vi "Path Keeper_User Find and Write.vi"(7 "Previous location":path, 8 "Error In":errorcluster, 9 "File(f)\nDirectory(t) In":bool, 10 "File / Directory Name In":string, 11 "Refnum In":T1) -> (0 "Error Out":errorcluster, 1 "Valid Path Out":bool, 2 "Path Out":path, 3 "Config Data Out":T1)   [LabVIEW 2015]
uses:
  <vilib>/Utility/config.llb/Config Data RefNum.ctl
  <vilib>/Utility/config.llb/NI_LVConfig.lvlib
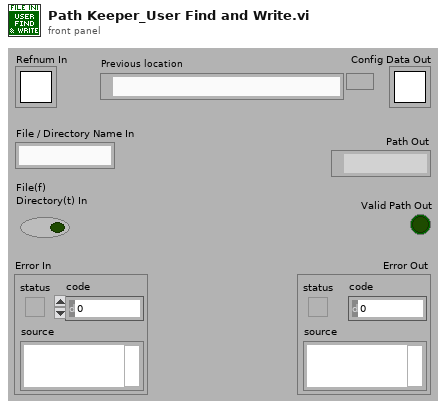
[diagram p1: front panel]
types:
  T1 = typedef "NI_LVConfig.lvlib/Config Data RefNum.ctl" = refnum<k1>
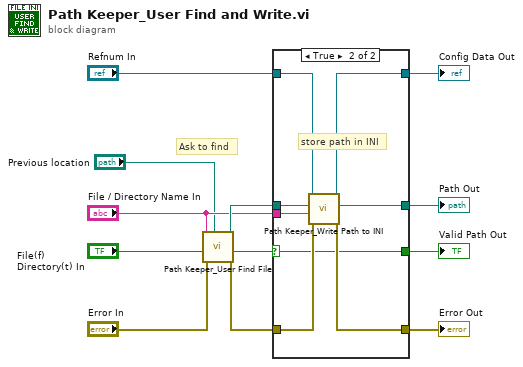
[diagram p0: block diagram]
diagram:
  # "Ask to find"
  n1 = call "Path Keeper_User Find File.vi"("Previous Path"="Previous location", "error In"="Error In", "File(f)\nDirectory(t) In"="File(f)\nDirectory(t) In", "File / Directory Name In"="File / Directory Name In") -> ("error Out"=w8:errorcluster, "Valid Item Out"=w10:bool, "path Out"=w4:path)  [unwired: 5 in]
  n2 = case shown="True" w10 {
    selector: w10 -> [w14 w16]
    tunnel: "File / Directory Name In" -> [_ w23]
    tunnel: w4 -> [_ w22]
    tunnel: "Refnum In" -> [w15 w21]
    tunnel: [w15 w20] -> w6
    tunnel: w8 -> [w13 w19]
    tunnel: [w13 w18] -> w9
    tunnel: [_ w17] -> w11
    tunnel: [w14 w16] -> w12
    frame False {
      # "No Path Found"
    }
    frame True {
      # "store path in INI"
      n3 = call "Path Keeper_Write Path to INI.vi"("Error In"=w19, "File / Directory Name In"=w23, "Path In"=w22, "Ini Ref In"=w21) -> ("Error Out"=w18:errorcluster, "Path Out"=w17:path, "Ini Ref Out"=w20:T1)  [unwired: 5 in]
    }
  }
  "Valid Path Out" <- w12
  "Path Out" <- w11
  "Error Out" <- w9
  "Config Data Out" <- w6
